vi "Test position.vi"() -> ()   [LabVIEW 2014]
uses:
  SerialController/Serial Controller.lvclass
panel:
  out "Position":dbl[](array[numeric])
  in  "VISA resource name":refnum<visa-resource-name>="COM2"
  in  "Serial Controller.lvclass":refnum<class "Serial Controller.lvclass">
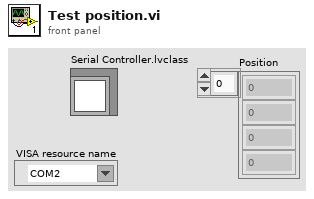
[diagram p1: front panel]
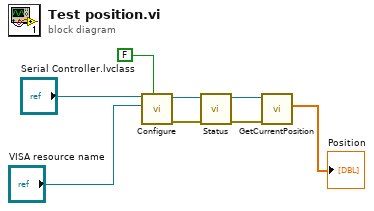
[diagram p0: block diagram]
diagram:
  n1 = call-dynamic "Configure.vi"("Reset"=FALSE, "VISA resource name"="VISA resource name", "Serial Controller in"="Serial Controller.lvclass") -> ("error out"=w3:errorcluster, "Serial Controller out"=w4:refnum<class "Serial Controller.lvclass">)  [unwired: 7 in]
  n2 = call-dynamic "Status.vi"("error in (no error)"=w3, "Serial Controller in"=w4) -> ("error out"=w2:errorcluster, "Serial Controller out"=w1:refnum<class "Serial Controller.lvclass">)  [unwired: 7 in, 1 out]
  n3 = call-dynamic "GetCurrentPosition.vi"("error in (no error)"=w2, "Serial Controller in"=w1) -> ("Position"=→"Position":dbl[])  [unwired: 6 in, 3 out]
